vi "Build Control Packet.vi"(8 "error in (no error)":errorcluster, 9 "Incoming Packets":u8[](array[numeric]) format="%08b", 11 "Incomplete ControlPacket":refnum<class "ControlPacket.lvclass">) -> (0 "error out":errorcluster, 1 "Remaining Packets":u8[](array[numeric]) format="%08b", 2 "Complete Packet":bool, 3 "ControlPacket":refnum<class "ControlPacket.lvclass">)   [LabVIEW 2013, in "ControlPacket.lvclass"]
uses:
  ControlPacket.lvclass
  ControlPacket.lvclass/ControlPacket.ctl
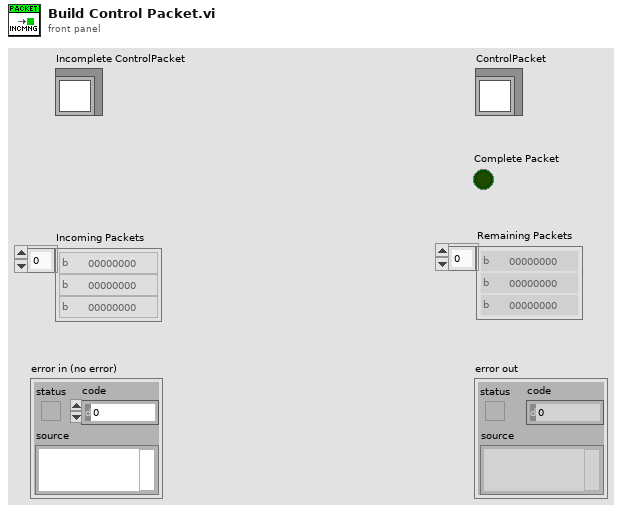
[diagram p1: front panel]
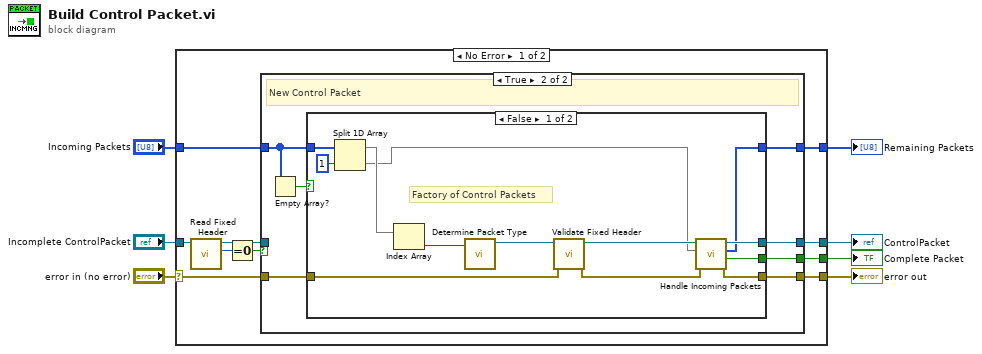
[diagram p0: block diagram]
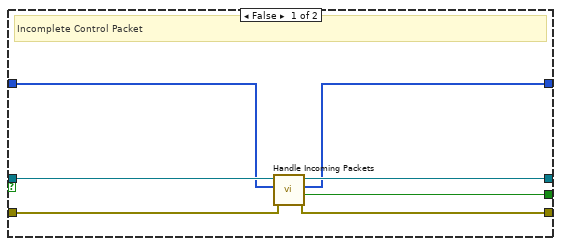
[diagram p2: hidden frame]
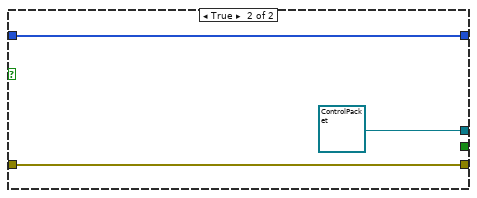
[diagram p3: hidden frame]
diagram:
  n1 = case shown="No Error" "error in (no error)" {
    selector: "error in (no error)" -> [w11 w50]
    tunnel: [w10 w50] -> w6
    tunnel: "Incomplete ControlPacket" -> [w17 w48]
    tunnel: "Incoming Packets" -> [w13 w49]
    tunnel: [w12 w48] -> w3
    tunnel: [w9 w49] -> w2
    tunnel: [w8 _] -> w1
    frame No Error {
      n2 = call "Read Fixed Header.vi"("ControlPacket in"=w17) -> ("Fixed Header"=w16:u8, "ControlPacket out"=w14:refnum<class "ControlPacket.lvclass">)  [unwired: 9 in]
      n3 = Equal To 0?(x=w16) -> (x = 0?=w15:bool)
      n4 = case shown="True" w15 {
        tunnel: w14 -> [w24 _]
        tunnel: w13 -> [w22 w26]
        tunnel: [w23 w30] -> w12
        tunnel: w11 -> [w20 w31]
        tunnel: [w19 w29] -> w10
        tunnel: [w21 w28] -> w9
        tunnel: [w18 w27] -> w8
        frame False {
          # "Incomplete Control Packet"
          n5 = call "Handle Incoming Packets.vi"("error in (no error)"=w20, "Incoming Packets"=w22, "ControlPacket in"=w24) -> ("error out"=w19:errorcluster, "Complete?"=w18:bool, "Remaining Packets"=w21:u8[], "ControlPacket out"=w23:refnum<class "ControlPacket.lvclass">)  [unwired: 5 in]
        }
        frame True {
          # "New Control Packet"
          n6 = Empty Array?(array=w26) -> (empty?=w25:bool)
          n7 = case shown="False" w25 {
            tunnel: w31 -> [w36 w46]
            tunnel: [w44 refnum<class "ControlPacket.lvclass"> refnum ("ControlPacket.lvclass")] -> w30
            tunnel: [w43 w46] -> w29
            tunnel: [w42 w47] -> w28
            tunnel: [w41 _] -> w27
            tunnel: w26 -> [w39 w47]
            frame False {
              # "Factory of Control Packets"
              n8 = Split 1D Array(array=w39, index=1 ("length")) -> (first subarray=w40:u8[], second subarray=w32:u8[])
              n9 = Index Array(array=w40) -> (element=w37:u8)  [unwired: 1 in]
              n10 = call "Determine Packet Type.vi"("Fixed Header"=w37) -> ("Packet Type"=w34:refnum<class "ControlPacket.lvclass">)  [unwired: 10 in]
              n11 = call-dynamic "Validate Fixed Header.vi"("error in (no error)"=w36, "ControlPacket in"=w34) -> ("error out"=w35:errorcluster, "ControlPacket out"=w33:refnum<class "ControlPacket.lvclass">)  [unwired: 7 in, 1 out]
              n12 = call "Handle Incoming Packets.vi"("error in (no error)"=w35, "Incoming Packets"=w32, "ControlPacket in"=w33) -> ("error out"=w43:errorcluster, "Complete?"=w41:bool, "Remaining Packets"=w42:u8[], "ControlPacket out"=w44:refnum<class "ControlPacket.lvclass">)  [unwired: 5 in]
            }
            frame True {
            }
          }
        }
      }
    }
    frame Error {
    }
  }
  "error out" <- w6
  "ControlPacket" <- w3
  "Complete Packet" <- w1
  "Remaining Packets" <- w2
